vi "fitParams2Cluster.vi"(0 "Experimental Variables":T1={"Pixel Size before binning (µm)"=6.0, "Imaging Wavelength (m)"=4.61e-07, "Isotope"=84, "1P1 Linewidth (MHz)"=30.5, "Imaging Detuning (MHz)"=0.0, "Software Bin Size"=1, "Exp. Trigger ON time (ms)"=0.0, "Path to spinapi.dll"=path "C:/SpinCore/SpinAPI/lib32/spinapi.dll", "PB clock_freq (MHz)"=100.0} {"Software Bin Size" items=["1"=1, "2"=2, "3"=3, "4"=4, "5"=5, "6"=6, "7"=7, "8"=8]; "Isotope" min=84 max=88; "Imaging Wavelength (m)" format="%#_6p"}, 1 "Best fit parameters":dbl[](array[numeric])) -> (7 "Best Fit Parameter Cluster":T2 {"Rot. Angle (deg)" format="%#.3g"; "Aspect Ratio" format="%#.3g"; "Y Width (um)" format="%#.3g"; "X Width (um)" format="%#.3g"; "Y Center (px)" format="%#.3g"; "X Center (px)" format="%#.3g"; "Amplitude (OD)" format="%#.3g"})   [LabVIEW 2016]
uses:
  Controls/2D Gaussian Fitting/Fit Parameter Cluster.ctl
  Controls/ExperimentParameters/experimentalvariables.ctl
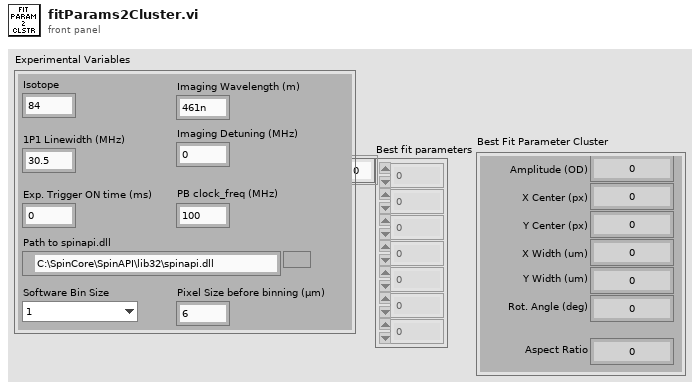
[diagram p1: front panel]
types:
  T1 = typedef "experimentalvariables.ctl" = cluster{"Pixel Size before binning (µm)":dbl, "Imaging Wavelength (m)":dbl, "Isotope":i32, "1P1 Linewidth (MHz)":dbl, "Imaging Detuning (MHz)":dbl, "Software Bin Size":u16, "Exp. Trigger ON time (ms)":dbl, "Path to spinapi.dll":path, "PB clock_freq (MHz)":dbl}
  T2 = typedef "Fit Parameter Cluster.ctl" = cluster{"Amplitude (OD)":dbl, "X Center (px)":dbl, "Y Center (px)":dbl, " X Width (um)":dbl, "Y Width (um)":dbl, "Aspect Ratio":dbl, "Rot. Angle (deg)":dbl}
  T3 = cluster{"Best fit parameters[0]":dbl, "Best fit parameters[1]":dbl, "Best fit parameters[2]":dbl, "Best fit parameters[3]":dbl, "Best fit parameters[4]":dbl, "Best fit parameters[5]":dbl, "Best fit parameters[6]":dbl, "Best fit parameters[7]":dbl, "Best fit parameters[8]":dbl}
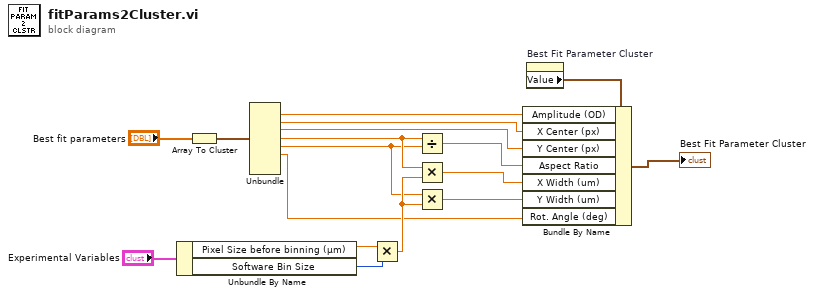
[diagram p0: block diagram]
diagram:
  n1 = Unbundle By Name("Experimental Variables") -> ("Pixel Size before binning (µm)"=w12:dbl, "Software Bin Size"=w13:u16)
  n2 = Array To Cluster(array="Best fit parameters") -> (cluster=w15:T3)
  n3 = Unbundle(w15) -> ("Best fit parameters[1]"=w6:dbl, "Best fit parameters[2]"=w5:dbl, "Best fit parameters[3]"=w4:dbl, "Best fit parameters[4]"=w3:dbl, "Best fit parameters[5]"=w2:dbl, "Best fit parameters[6]"=w1:dbl)  [unwired: 3 out]
  n4 = Multiply(x=w12, y=w13) -> (x*y=w9:dbl)
  n5 = Divide(x=w3, y=w2) -> (x/y=w10:dbl)
  n6 = Multiply(x=w3, y=w9) -> (x*y=w8:dbl)
  n7 = Multiply(x=w2, y=w9) -> (x*y=w7:dbl)
  n8 = property on="Best Fit Parameter Cluster" class="Clust (strict)"() -> ("Value"=w11:T2)  [unwired: 2 in, 2 out]
  n9 = Bundle By Name(cluster=w11, "Amplitude (OD)"=w6, "X Center (px)"=w5, "Y Center (px)"=w4, "Aspect Ratio"=w10, "X Width (um)"=w8, "Y Width (um)"=w7, "Rot. Angle (deg)"=w1) -> (→"Best Fit Parameter Cluster":T2)
